vi "Delete_Special_Case_Track(101-Empty)-1.vi"(4 "[IN] Special case!":bool, 5 "error IN":errorcluster, 6 "[IN] Subtracks":T1(array[cluster]), 7 "[IN] Cost function":i8[](array[numeric]), 8 "[IN] Clusters for Re\nconstructed Tracks":T2) -> (0 "error OUT":errorcluster, 3 "[OUT] Clusters for Re\nconstructed Tracks":T2)   [LabVIEW 2013]
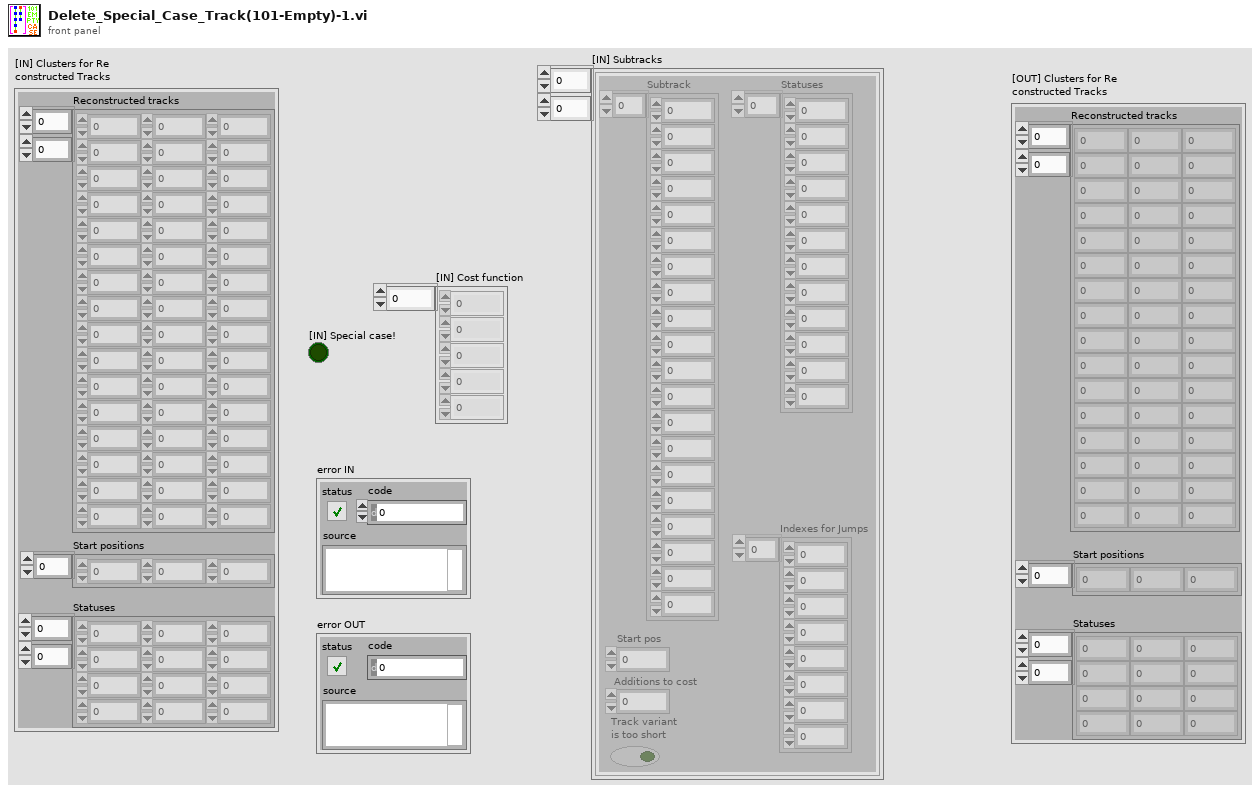
[diagram p1: front panel]
types:
  T1 = cluster{"Subtrack":dbl[], "Statuses":i16[], "Start pos":i32, "Additions to cost":i32, "Track variant \nis too short":bool, "Indexes for Jumps":i32[]}[][]
  T2 = cluster{"Reconstructed tracks":dbl[][], "Start positions":i32[], "Statuses":i16[][]}
  T3 = cluster{"Subtrack":dbl[], "Statuses":i16[], "Start pos":i32, "Additions to cost":i32, "Track variant \nis too short":bool, "Indexes for Jumps":i32[]}[]
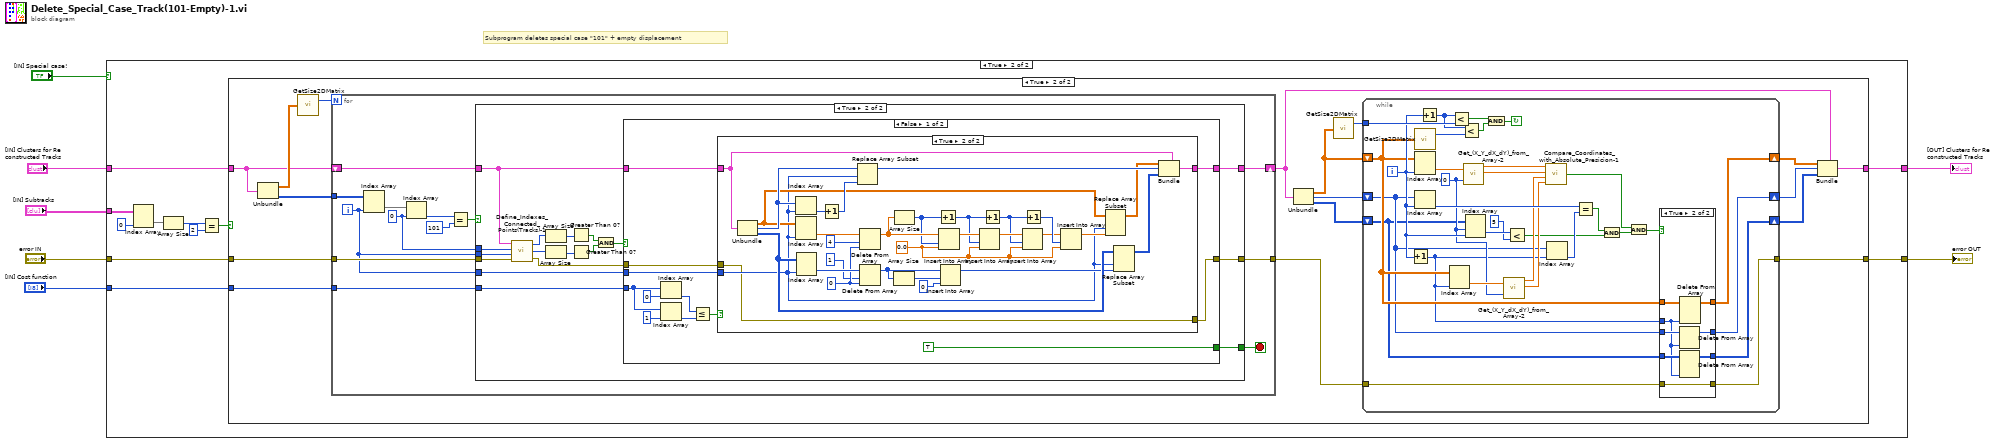
[diagram p0: block diagram]
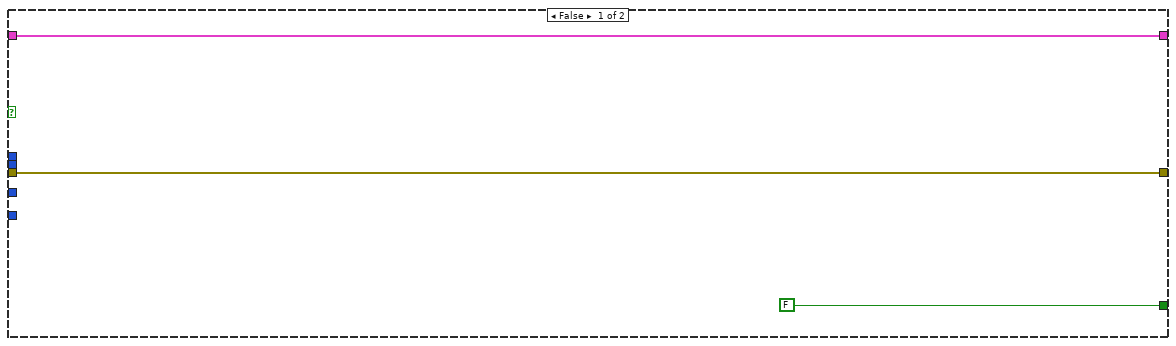
[diagram p5: hidden frame]
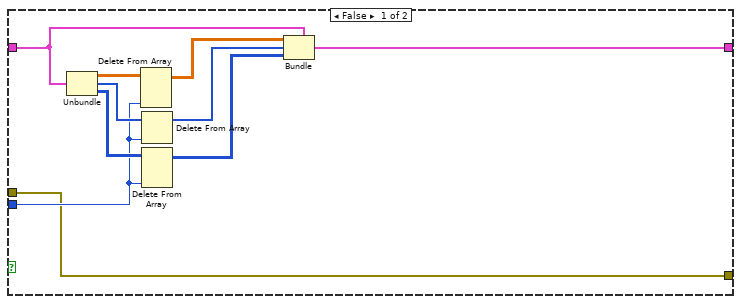
[diagram p6: hidden frame]
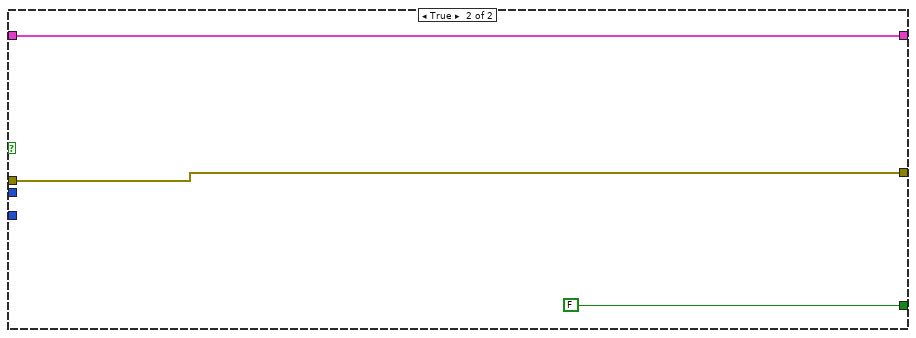
[diagram p7: hidden frame]
diagram:
  # "Subprogram deletes special case \"101\" + empty displacement"
  n1 = case shown="True" "[IN] Special case!" {
    tunnel: "[IN] Clusters for Re\nconstructed Tracks" -> [w9 w13]
    tunnel: "error IN" -> [w8 w12]
    tunnel: "[IN] Subtracks" -> [_ w20]
    tunnel: "[IN] Cost function" -> [_ w14]
    tunnel: [w9 w11] -> w2
    tunnel: [w8 w10] -> w1
    frame False {
    }
    frame True {
      n2 = Index Array(array=w20, index (col)=0 ("disabled index (col)")) -> (element=w18:T3)  [unwired: 1 in]
      n3 = Array Size(array=w18) -> (size(s)=w17:i32)
      n4 = Equal?(x=w17, y=2) -> (x = y?=w15:bool)
      n5 = case shown="True" w15 {
        tunnel: w14 -> [_ w34]
        tunnel: w13 -> [w22 w36]
        tunnel: w12 -> [w21 w35]
        tunnel: [w22 w25] -> w11
        tunnel: [w21 w28] -> w10
        frame False {
        }
        frame True {
          n6 = Unbundle(w36) -> ("Reconstructed tracks"=w39:dbl[][], "Statuses"=w37:i16[][])  [unwired: 1 out]
          n7 = call "GetSize2DMatrix.vi"("Array IN (2D)"=w39) -> ("# Cols"=w38:i32)  [unwired: 1 out]
          n8 = for {
            N: w38 -> [_]
            tunnel: w37 -> [w96]
            shift-right: [w87] -> w27
            shift-left: w36 -> [w91]
            tunnel: w35 -> [w90]
            tunnel: w34 -> [w88]
            tunnel: [w84] -> w29
            i -> [w86]
            stop <- w85 stop-if-true
            w89 = 0 ("index")
            n9 = Index Array(array=w96, index (col)=w86) -> (element=w95:i16[])  [unwired: 1 in]
            n10 = Index Array(array=w95, index=w89) -> (element=w94:i16)
            n11 = Equal?(x=w94, y=i16 101) -> (x = y?=w92:bool)
            n12 = case shown="True" w92 {
              tunnel: w91 -> [w98 w105]
              tunnel: w90 -> [w97 w116]
              tunnel: w89 -> [_ w115]
              tunnel: w86 -> [_ w114]
              tunnel: w88 -> [_ w106]
              tunnel: [w98 w104] -> w87
              tunnel: w86 -> [_ w103]
              tunnel: [FALSE w102] -> w85
              tunnel: [w97 w100] -> w84
              frame False {
              }
              frame True {
                n13 = call "Define_Indexes_Connected_Points(Tracks)-1.vi"("error IN"=w116, "[IN] Index of track with\n(problem displacement)"=w114, "[IN]Index of problem\ndisplacement inside track"=w115, "[IN] Track group"=w105) -> ("error OUT"=w101:errorcluster, "[OUT] Index of \nconnected dots\ninside the track"=w112:i32[], "[OUT] Index of connected\ntracks with problem dot"=w113:i32[])
                n14 = Array Size(array=w113) -> (size(s)=w111:i32)
                n15 = Array Size(array=w112) -> (size(s)=w110:i32)
                n16 = Greater Than 0?(x=w111) -> (x > 0?=w109:bool)
                n17 = Greater Than 0?(x=w110) -> (x > 0?=w108:bool)
                n18 = And(x=w109, y=w108) -> (x .and. y?=w107:bool)
                n19 = case shown="False" w107 {
                  tunnel: w106 -> [w127 _]
                  tunnel: w105 -> [w122 w172]
                  tunnel: [w120 w172] -> w104
                  tunnel: w103 -> [w121 _]
                  tunnel: [TRUE FALSE] -> w102
                  tunnel: w101 -> [w118 w170]
                  tunnel: [w117 w170] -> w100
                  frame False {
                    n20 = Index Array(array=w127, index=0) -> (element=w125:i8)
                    n21 = Index Array(array=w127, index=1) -> (element=w124:i8)
                    n22 = Less Or Equal?(x=w125, y=w124) -> (x <= y?=w123:bool)
                    n23 = case shown="True" w123 {
                      tunnel: w122 -> [w134 w150]
                      tunnel: w121 -> [w135 w141]
                      tunnel: [w133 w151] -> w120
                      tunnel: w118 -> [w129 w139]
                      tunnel: [w129 w139] -> w117
                      frame False {
                        n24 = Unbundle(w134) -> ("Reconstructed tracks"=w138:dbl[][], "Start positions"=w137:i32[], "Statuses"=w136:i16[][])
                        n25 = Delete From Array(array=w138, index (col)=w135) -> (array with subset deleted=w132:dbl[][])  [unwired: 2 in, 1 out]
                        n26 = Delete From Array(array=w137, index=w135) -> (array with subset deleted=w131:i32[])  [unwired: 1 in, 1 out]
                        n27 = Delete From Array(array=w136, index (col)=w135) -> (array with subset deleted=w130:i16[][])  [unwired: 2 in, 1 out]
                        n28 = Bundle(cluster=w134, "Reconstructed tracks"=w132, "Start positions"=w131, "Statuses"=w130) -> (w133:T2)
                      }
                      frame True {
                        w155 = 0.0 ("new element/subarray")
                        w165 = 0 ("index")
                        n29 = Unbundle(w150) -> ("Reconstructed tracks"=w146:dbl[][], "Start positions"=w149:i32[], "Statuses"=w143:i16[][])
                        n30 = Index Array(array=w149, index=w141) -> (element=w169:i32)
                        n31 = Index Array(array=w146, index (col)=w141) -> (element=w168:dbl[])  [unwired: 1 in]
                        n32 = Index Array(array=w143, index (col)=w141) -> (element=w166:i16[])  [unwired: 1 in]
                        n33 = Increment(x=w169) -> (x+1=w148:i32)
                        n34 = Replace Array Subset(array=w149, new element=w148, index=w141) -> (w147:i32[])
                        n35 = Delete From Array(array=w168, length=4, index=w165) -> (array with subset deleted=w163:dbl[])  [unwired: 1 out]
                        n36 = Delete From Array(array=w166, length=1, index=w165) -> (array with subset deleted=w154:i16[])  [unwired: 1 out]
                        n37 = Array Size(array=w154) -> (size(s)=w153:i32)
                        n38 = Array Size(array=w163) -> (size(s)=w161:i32)
                        n39 = Increment(x=w161) -> (x+1=w160:i32)
                        n40 = Insert Into Array(array=w163, index=w161, new element=w155) -> (w162:dbl[])
                        n41 = Insert Into Array(array=w154, index=w153, new element=i16 0 ("new element/subarray")) -> (w142:i16[])
                        n42 = Insert Into Array(array=w162, index=w160, new element=w155) -> (w159:dbl[])
                        n43 = Increment(x=w160) -> (x+1=w158:i32)
                        n44 = Insert Into Array(array=w159, index=w158, new element=w155) -> (w156:dbl[])
                        n45 = Increment(x=w158) -> (x+1=w157:i32)
                        n46 = Insert Into Array(array=w156, index=w157, new element=w155) -> (w145:dbl[])
                        n47 = Replace Array Subset(array=w146, new element=w145, index (col)=w141) -> (w144:dbl[][])  [unwired: 1 in]
                        n48 = Replace Array Subset(array=w143, new element=w142, index (col)=w141) -> (w140:i16[][])  [unwired: 1 in]
                        n49 = Bundle(cluster=w150, "Reconstructed tracks"=w144, "Start positions"=w147, "Statuses"=w140) -> (w151:T2)
                      }
                    }
                  }
                  frame True {
                  }
                }
              }
            }
          }
          n50 = Unbundle(w27) -> ("Reconstructed tracks"=w32:dbl[][], "Start positions"=w30:i32[], "Statuses"=w31:i16[][])
          n51 = call "GetSize2DMatrix.vi"("Array IN (2D)"=w32) -> ("# Cols"=w33:i32)  [unwired: 1 out]
          n52 = while {
            tunnel: w33 -> [w68]
            shift-right: [w47] -> w26
            shift-left: w32 -> [w48]
            shift-right: [w45] -> w24
            shift-left: w30 -> [w46]
            shift-right: [w42] -> w23
            shift-left: w31 -> [w44]
            tunnel: w29 -> [w41]
            tunnel: [w40] -> w28
            i -> [w62]
            stop <- w63 continue-if-true
            w57 = 0 ("Index of Displacement")
            n53 = Increment(x=w62) -> (x+1=w43:i32)
            n54 = call "GetSize2DMatrix.vi"("Array IN (2D)"=w48) -> ("# Cols"=w65:i32)  [unwired: 1 out]
            n55 = Index Array(array=w48, index (col)=w62) -> (element=w71:dbl[])  [unwired: 1 in]
            n56 = Index Array(array=w46, index=w62) -> (element=w59:i32)
            n57 = Increment(x=w62) -> (x+1=w66:i32)
            n58 = Index Array(array=w48, index (col)=w43) -> (element=w58:dbl[])  [unwired: 1 in]
            n59 = Less?(x=w66, y=w68) -> (x < y?=w67:bool)
            n60 = Less?(x=w66, y=w65) -> (x < y?=w64:bool)
            n61 = call "Get_(X_Y_dX_dY)_from_Array-2.vi"("(X,Y,dX,dY)"=w71, "Index of Displacement"=w57) -> ("X"=w70:dbl, "Y"=w69:dbl)  [unwired: 2 out]
            n62 = Index Array(array=w44, index (row)=w57, index (col)=w62) -> (element=w61:i16)
            n63 = And(x=w67, y=w64) -> (x .and. y?=w63:bool)
            n64 = call "Get_(X_Y_dX_dY)_from_Array-2.vi"("(X,Y,dX,dY)"=w58, "Index of Displacement"=w57) -> ("X"=w56:dbl, "Y"=w55:dbl)  [unwired: 2 out]
            n65 = Less?(x=w61, y=i16 5) -> (x < y?=w53:bool)
            n66 = call "Compare_Coordinates_with_Absolute_Presicion-1.vi"("X 1"=w70, "Y 1"=w69, "X 2"=w56, "Y 2"=w55) -> ("[OUT] Same coordinates?"=w51:bool)  [unwired: 1 in]
            n67 = Index Array(array=w46, index=w43) -> (element=w54:i32)
            n68 = Equal?(x=w59, y=w54) -> (x = y?=w52:bool)
            n69 = And(x=w52, y=w53) -> (x .and. y?=w50:bool)
            n70 = And(x=w51, y=w50) -> (x .and. y?=w49:bool)
            n71 = case shown="True" w49 {
              tunnel: w48 -> [w75 w83]
              tunnel: w43 -> [_ w78]
              tunnel: [w75 w82] -> w47
              tunnel: w46 -> [w74 w81]
              tunnel: [w74 w80] -> w45
              tunnel: w44 -> [w73 w79]
              tunnel: [w73 w77] -> w42
              tunnel: w41 -> [w72 w76]
              tunnel: [w72 w76] -> w40
              frame False {
              }
              frame True {
                n72 = Delete From Array(array=w81, index=w78) -> (array with subset deleted=w80:i32[])  [unwired: 1 in, 1 out]
                n73 = Delete From Array(array=w79, index (col)=w78) -> (array with subset deleted=w77:i16[][])  [unwired: 2 in, 1 out]
                n74 = Delete From Array(array=w83, index (col)=w78) -> (array with subset deleted=w82:dbl[][])  [unwired: 2 in, 1 out]
              }
            }
          }
          n75 = Bundle(cluster=w27, "Reconstructed tracks"=w26, "Start positions"=w24, "Statuses"=w23) -> (w25:T2)
        }
      }
    }
  }
  "[OUT] Clusters for Re\nconstructed Tracks" <- w2
  "error OUT" <- w1
